vi "OAT Tachless Globa Settings.vi"() -> ()   [LabVIEW 2017, in "SoundVib_Tachless.lvlib"]
uses:
  <vilib>/addons/Sound and Vibration/Order Analysis/Tachless/SoundVib_Tachless.lvlib
panel:
  in  "Default Mask \nWidth (Pixels)":i32=3
  in  "Current Order":dbl=1.0 format="%.2f"
  in  "Default Points":i32=5
  in  "Window Length":T1(ring)
  # "JTFA"
  # "Initiate"
  # "Refine"
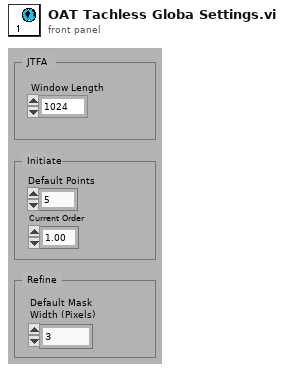
[diagram p1: front panel]
types:
  T1 = enum16{"1024", "2048", "4096", "8192", "16384", "32768"}
diagram:
